vi "Write Specific&CommonTriggerProperties.vi"(8 "error in (no error)":errorcluster, 10 "Specific&CommonTriggerProperties":T1={"Common Trigger Settings"={"Trigger Delay"=0.0, "Reference Position"=50.0, "Trigger Modifier"=2, "Auto Triggered"=FALSE}, "Specific Trigger Settings"={"Source"="", "Holdoff"=0.0, "Level"=0.0, "Trigger Slope"=enum."Negative", "Type"=enum."Immediate", "Window Mode"=0, "Low Level"=-0.1, "High Level"=0.1, "Coupling"=1, "Hysteresis"=0.05}} {"Specific Trigger Settings"."Hysteresis" format="%.2f"; "Specific Trigger Settings"."Coupling" items=["AC"=0, "DC"=1, "HF Reject"=3, "LF Reject"=4, "AC Plus HF Reject"=1001]; "Specific Trigger Settings"."High Level" format="%.2f"; "Specific Trigger Settings"."Low Level" format="%.2f"; "Specific Trigger Settings"."Window Mode" items=["Entering", "Leaving"]; "Common Trigger Settings"."Trigger Modifier" items=["None"=1, "Auto Trigger"=2]; "Common Trigger Settings"."Reference Position" format="%.1f"; "Common Trigger Settings"."Trigger Delay" format="%#.4p"}, 11 "ScopePluginsBase in":refnum<class "ScopePluginsBase.lvclass">) -> (0 "error out":errorcluster, 3 "ScopePluginsBase out":refnum<class "ScopePluginsBase.lvclass">)   [LabVIEW 2018, in "ScopePlugins.lvlib" / "ScopePluginsBase.lvclass"]
uses:
  ScopePluginsBase.lvclass
  Typedefs/TriggerSettings.ctl
  ScopePluginsBase.lvclass/ScopePluginsBase.ctl
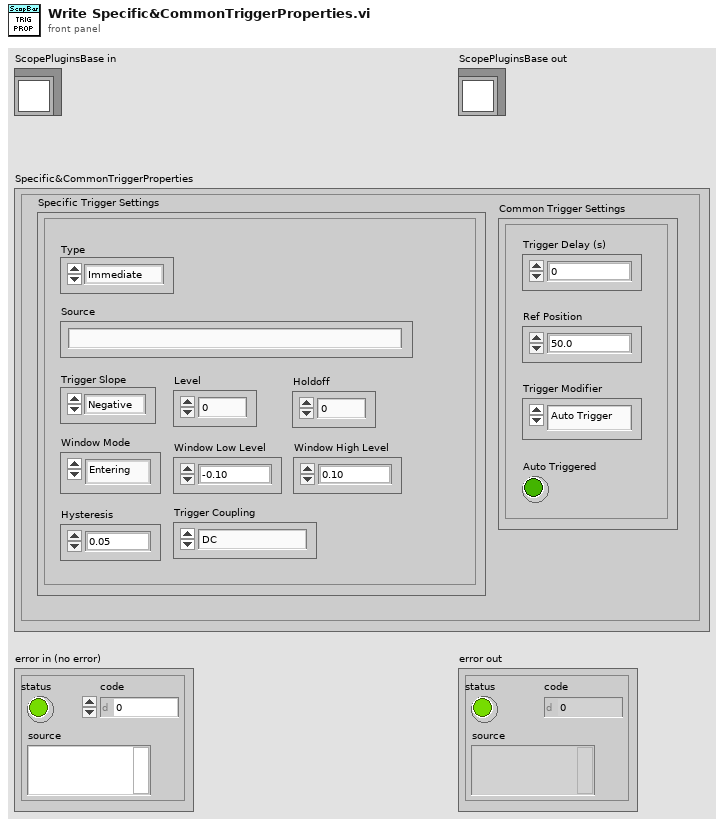
[diagram p1: front panel]
types:
  T1 = typedef "ScopePlugins.lvlib/ScopePluginsBase.lvclass/TriggerSettings.ctl" = cluster{"Common Trigger Settings":cluster{"Trigger Delay":dbl, "Reference Position":dbl, "Trigger Modifier":i32, "Auto Triggered":bool}, "Specific Trigger Settings":cluster{"Source":string, "Holdoff":dbl, "Level":dbl, "Trigger Slope":enum16{"Negative", "Positive"}, "Type":enum16{"Immediate", "Edge", "Digitial", "Window", "Hysteresis", "Width", "Runt", "Glitch", "TV", "AC Line"}, "Window Mode":i32, "Low Level":dbl, "High Level":dbl, "Coupling":u16, "Hysteresis":dbl}}
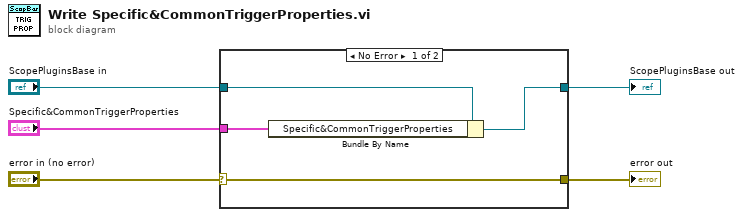
[diagram p0: block diagram]
diagram:
  n1 = case shown="No Error" "error in (no error)" {
    selector: "error in (no error)" -> [w9 w10]
    tunnel: [w9 w10] -> w4
    tunnel: [w7 w11] -> w2
    tunnel: "ScopePluginsBase in" -> [w8 w11]
    tunnel: "Specific&CommonTriggerProperties" -> [w6 _]
    frame No Error {
      n2 = Bundle By Name(cluster=w8, "Specific&CommonTriggerProperties"=w6) -> (w7:refnum<class "ScopePluginsBase.lvclass">)
    }
    frame Error {
    }
  }
  "error out" <- w4
  "ScopePluginsBase out" <- w2
